vi "Is this panel cloneable.vi"(8 "error in (no error)":errorcluster, 11 "Fiber Auto Collimation panel in":refnum<class "Fiber Auto Collimation panel.lvclass">) -> (0 "error out":errorcluster, 2 "This class is cloneable":bool, 3 "Fiber Auto Collimation panel out":refnum<class "Fiber Auto Collimation panel.lvclass">)   [LabVIEW 2018, in "Fiber Auto Collimation panel.lvclass"]
doc: "Returns True if the class wire calling this VI is one that can launch multiple front panels.\n\nThis VI always returns False if calling the top level class or any class that doesn't override it. Any class that is always or conditionally clonable should create an override for this VI that returns True either always or conditionally."
uses:
  Fiber Auto Collimation panel.lvclass
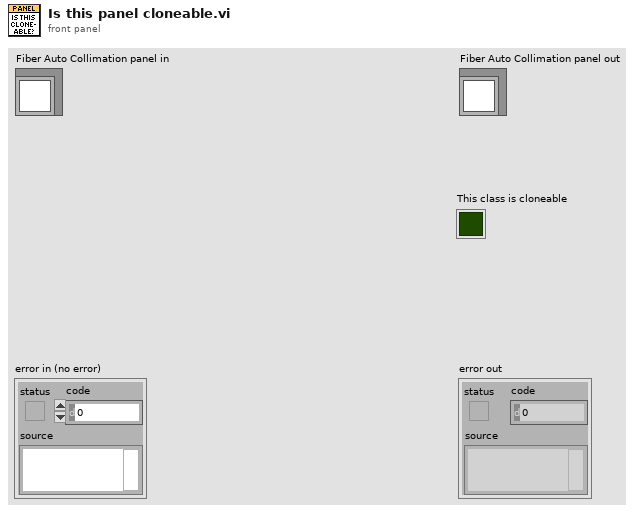
[diagram p1: front panel]
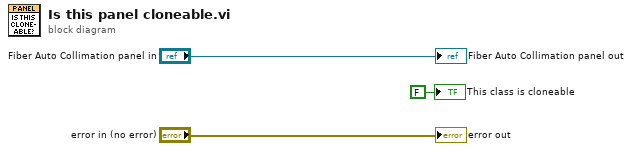
[diagram p0: block diagram]
diagram:
  "error out" <- "error in (no error)"
  "Fiber Auto Collimation panel out" <- "Fiber Auto Collimation panel in"
  "This class is cloneable" <- FALSE ("This class is cloneable")
